vi "hse-application_DetermineConfigAndDataDirectories.vi"(8 "error in (no error)":errorcluster, 10 "Application Directory":path, 11 "Application Name":string) -> (0 "error out":errorcluster, 2 "Data Directory":path, 3 "Config Directory":path)   [LabVIEW 2014, in "hse-application.lvclass"]
doc: "Determines the paths of the _Config and _Data directories: \n- either by reading from the [HSE] section of <%APPNAME%>.ini in the application directory\n- or by defining them to live parallel to the application directory (this is HSE default)"
uses:
  hse-application.lvclass
  hse-configuration/hse-config-ini/hse-config-ini.lvclass
  hse-configuration/hse-config-ini/hse-config-ini_ConfigData.ctl
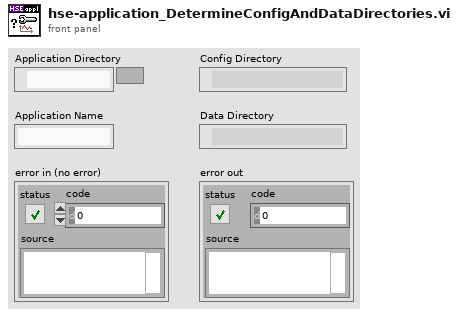
[diagram p1: front panel]
types:
  T1 = typedef "hse-config-ini.lvclass/hse-config-ini_ConfigData.ctl" = cluster{"Path to .ini file":path}
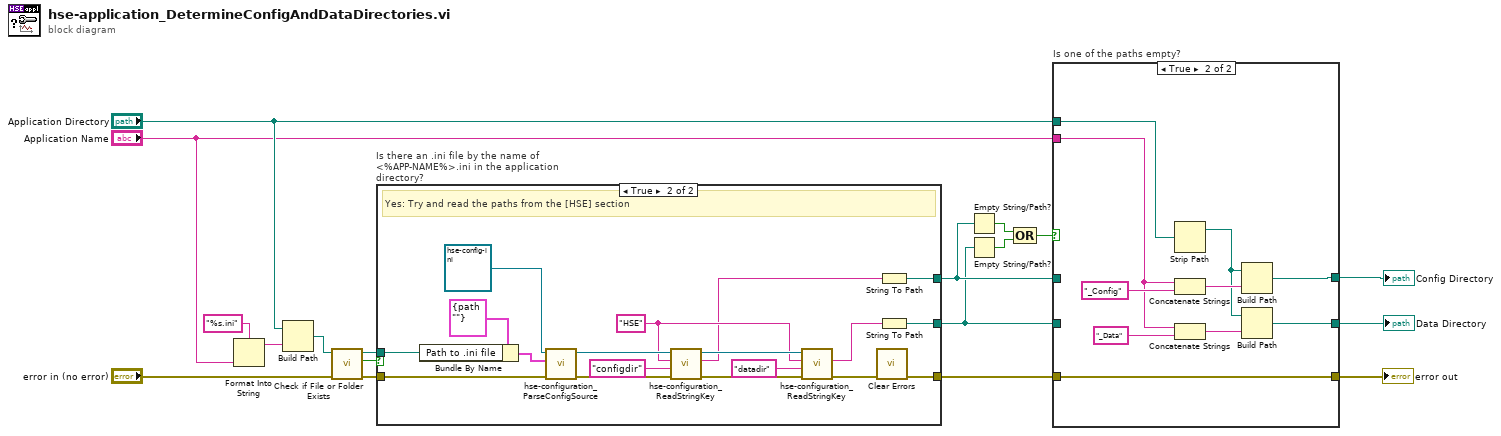
[diagram p0: block diagram]
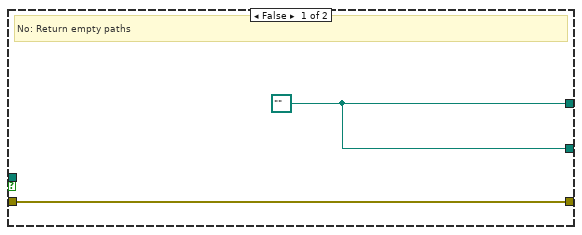
[diagram p3: hidden frame]
diagram:
  n1 = Format Into String(format string="%s.ini", "Application Name") -> (resulting string=w16:string)  [unwired: 2 in, 1 out]
  n2 = Build Path(base path="Application Directory", name or relative path=w16) -> (appended path=w15:path)
  n3 = call <vilib>:"Check if File or Folder Exists.vi"("error in (no error)"="error in (no error)", "path"=w15) -> ("error out"=w12:errorcluster, "file or folder exists?"=w14:bool, "dup path"=w13:path)  [unwired: 7 in]
  n4 = case "Is there an .ini file by the name of <%APP-NAME%>.ini in the application directory?" shown="True" w14 {
    tunnel: [w20 w23] -> w4
    tunnel: [w20 w24] -> w6
    tunnel: w13 -> [_ w26]
    tunnel: w12 -> [w19 w27]
    tunnel: [w19 w21] -> w2
    frame False {
      w20 = path "" ("appended path")
      # "No: Return empty paths"
    }
    frame True {
      w29 = "HSE" ("Section")
      # "Yes: Try and read the paths from the [HSE] section"
      n5 = Bundle By Name(cluster=T1 {"Path to .ini file"=path ""} ("Config Data"), "Path to .ini file"=w26) -> (w38:T1)
      n6 = call-dynamic "hse-configuration_ParseConfigSource.vi"("error in (no error)"=w27, "Config Source"=w38, "hse-config-ini in"=refnum<class "hse-config-ini.lvclass"> refnum ("hse-config-ini.lvclass")) -> ("error out"=w34:errorcluster, "hse-config-ini out"=w35:refnum<class "hse-config-ini.lvclass">)  [unwired: 7 in]
      n7 = call-dynamic "hse-configuration_ReadStringKey.vi"("error in (no error)"=w34, "Key"="configdir", "Section"=w29, "hse-config-ini in"=w35) -> ("error out"=w30:errorcluster, "Value"=w25:string, "hse-config-ini out"=w31:refnum<class "hse-config-ini.lvclass">)  [unwired: 5 in]
      n8 = call-dynamic "hse-configuration_ReadStringKey.vi"("error in (no error)"=w30, "Key"="datadir", "Section"=w29, "hse-config-ini in"=w31) -> ("error out"=w22:errorcluster, "Value"=w28:string)  [unwired: 5 in, 1 out]
      n9 = call <vilib>:"Clear Errors.vi"("error in (no error)"=w22) -> ("error out"=w21:errorcluster)  [unwired: 5 in, 1 out]
      n10 = String To Path(string=w25) -> (path=w24:path)
      n11 = String To Path(string=w28) -> (path=w23:path)
    }
  }
  n12 = Empty String/Path?(string/path=w6) -> (empty?=w9:bool)
  n13 = Empty String/Path?(string/path=w4) -> (empty?=w8:bool)
  n14 = Compound Arithmetic op=OR(w9, w8) -> (w7:bool)
  n15 = case "Is one of the paths empty?" shown="True" w7 {
    tunnel: "Application Directory" -> [_ w42]
    tunnel: "Application Name" -> [_ w46]
    tunnel: [w41 w45] -> w5
    tunnel: w6 -> [w41 _]
    tunnel: [w40 w44] -> w3
    tunnel: w4 -> [w40 _]
    tunnel: w2 -> [w39 w43]
    tunnel: [w39 w43] -> w1
    frame False {
    }
    frame True {
      n16 = Strip Path(path=w42) -> (stripped path=w48:path)  [unwired: 1 out]
      n17 = Concatenate Strings(w46, "_Config" ("Substring")) -> (w49:string)
      n18 = Concatenate Strings(w46, "_Data" ("Substring")) -> (w47:string)
      n19 = Build Path(base path=w48, name or relative path=w49) -> (appended path=w45:path)
      n20 = Build Path(base path=w48, name or relative path=w47) -> (appended path=w44:path)
    }
  }
  "error out" <- w1
  "Data Directory" <- w3
  "Config Directory" <- w5
